vi "tc_alarm.vi"(11 "alarm":i32) -> (3 "Status":string)   [LabVIEW 2017]
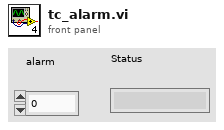
[diagram p1: front panel]
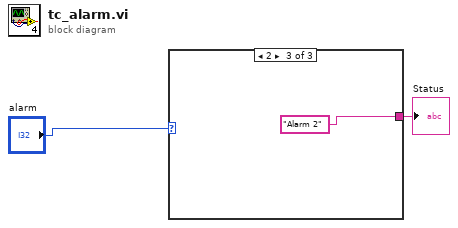
[diagram p0: block diagram]
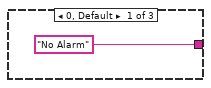
[diagram p2: hidden frame]
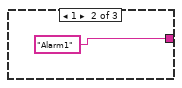
[diagram p3: hidden frame]
diagram:
  n1 = case shown="2" "alarm" {
    tunnel: ["No Alarm" "Alarm1" "Alarm 2"] -> w1
    frame 0, Default {
    }
    frame 1 {
    }
    frame 2 {
    }
  }
  "Status" <- w1
